vi "Get RGB Gains.vi"(8 "Error In":errorcluster, 11 "Display In":refnum<class "Display.lvclass">) -> (0 "Error Out":errorcluster, 2 "RGB Gains":T1, 3 "Display Out":refnum<class "Display.lvclass">)   [LabVIEW 2019, in "Display.lvclass"]
uses:
  Display.lvclass
  Public/Controls/RGB Gains.ctl
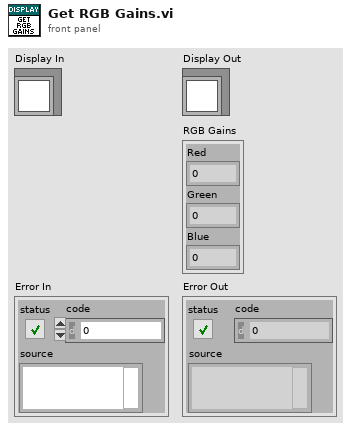
[diagram p1: front panel]
types:
  T1 = typedef "Display.lvclass/RGB Gains.ctl" = cluster{"Red":sgl, "Green":sgl, "Blue":sgl}
  T2 = typedef "Display.lvclass/Data.ctl" = cluster{"Size":T3, "Display Elements":refnum<class "Display Element.lvclass">[], "Frame":u32[][], "RGB Gains":T1}
  T3 = typedef "Display.lvclass/Size.ctl" = cluster{"Width":i32, "Height":i32}
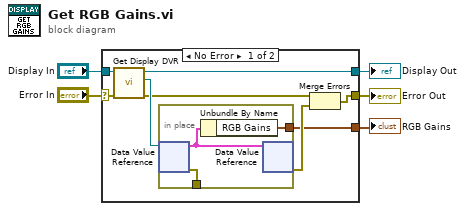
[diagram p0: block diagram]
diagram:
  n1 = case shown="No Error" "Error In" {
    selector: "Error In" -> [w9 w17]
    tunnel: [w11 w17] -> w2
    tunnel: [w8 w18] -> w1
    tunnel: "Display In" -> [w10 w18]
    tunnel: [w12 _] -> w3
    frame No Error {
      n2 = call "Get Display DVR.vi"("Error In"=w9, "Display In"=w10) -> ("Error Out"=w6:errorcluster, "DVR"=w7:refnum<data-value>, "Display Out"=w8:refnum<class "Display.lvclass">)  [unwired: 7 in]
      n3 = in-place {
        in-place-border: [w14] -> w12
        in-place-border: [w16] -> _
        n4 = in-place-dvr #1(w7) -> (w15:T2, w16:errorcluster)
        n5 = Unbundle By Name(w15) -> ("RGB Gains"=w14:T1)
        n6 = in-place-dvr #1(w15) -> (w13:errorcluster)  [unwired: 1 out]
      }
      n7 = Merge Errors(w6, w13) -> (w11:errorcluster)
    }
    frame Error {
    }
  }
  "Display Out" <- w1
  "Error Out" <- w2
  "RGB Gains" <- w3
